vi "Rapidox read.vi"() -> (2 "Output":u8[](array[numeric]))   [LabVIEW 2014]
uses:
  <vilib>/rvi/eio/common/nirviEmuTemplateMethod_errors.vi
  <vilib>/eio/EIOMethodNode/EIOMethodNode.xnode
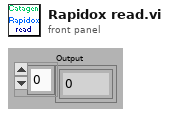
[diagram p1: front panel]
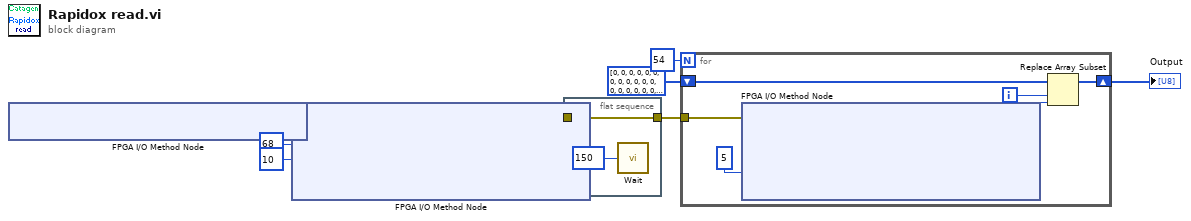
[diagram p0: block diagram]
diagram:
  n1 = xnode "FPGA I/O Method Node"() -> ("error out"=w3:errorcluster)  [unwired: 2 in, 1 out]
  n2 = xnode "FPGA I/O Method Node"("error in"=w3, "Data"=u8 68, "Timeout (ms)"=10) -> ("error out"=w2:errorcluster)  [unwired: 1 in, 2 out]
  n3 = flat-sequence {
    tunnel: w2 -> [w10]
    tunnel: [w10] -> w1
    frame #0 {
      n4 = call "Wait"("Count(mSec)"=u32 150) -> ()  [unwired: 1 out]
    }
  }
  n5 = for {
    N: 54 -> [_]
    tunnel: w1 -> [w16]
    shift-right: [w12] -> w5
    shift-left: u8[] [0, 0, 0, 0, 0, 0, 0, 0, 0, 0, 0, 0, 0, 0, 0, 0, 0, 0, 0, 0, 0, 0, 0, 0, 0, 0, 0, 0, 0, 0, 0, 0, 0, 0, 0, 0, 0, 0, 0, 0, 0, 0, 0, 0, 0, 0, 0, 0, 0, 0, 0, 0, 0, 0] -> [w14]
    i -> [w11]
    n6 = xnode "FPGA I/O Method Node"("error in"=w16, "Timeout (ms)"=5) -> ("Data"=w13:u8)  [unwired: 1 in, 3 out]
    n7 = Replace Array Subset(array=w14, new element=w13, index=w11) -> (w12:u8[])
  }
  "Output" <- w5
